vi "PI_Line_Scan_Prepare.vi"(0 "Pixel":u16=100, 3 "Line Length":dbl=20.0 min=0.1 max=200.0 format="%1.1f um", 5 "Wave Cycles":u16, 7 "Axis":enum32{"x-Axis", "y-Axis", "z-Axis"}(ring), 9 "Scanner Divider":i32) -> (14 "Commandset out":string[](array[string]), 16 "Measurement time / [s]":dbl)   [LabVIEW 2011]
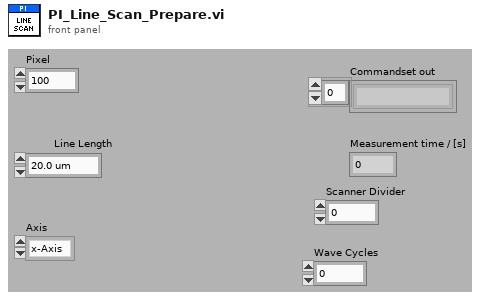
[diagram p1: front panel]
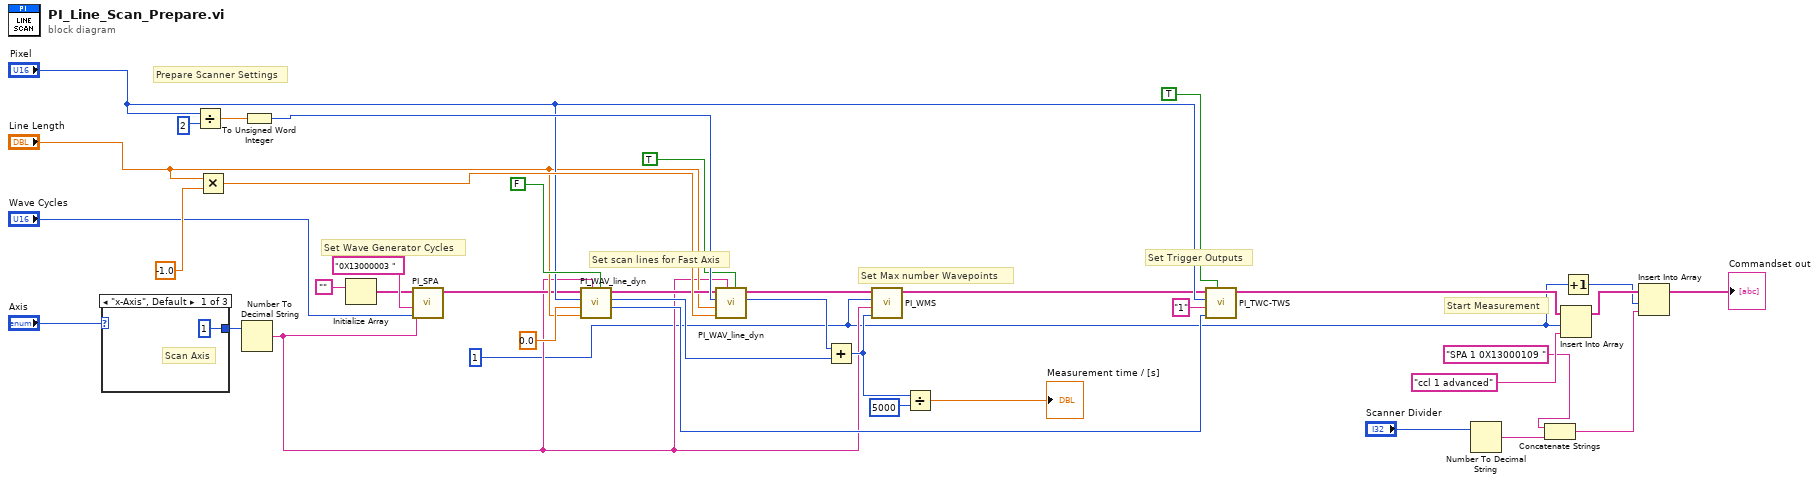
[diagram p0: block diagram]
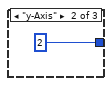
[diagram p2: hidden frame]
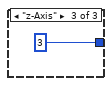
[diagram p3: hidden frame]
diagram:
  w7 = 1 ("Position / Commandset")
  # "Set Wave Generator Cycles"
  # "Start Measurement"
  # "Set Trigger Outputs"
  # "Set Max number Wavepoints"
  # "Set scan lines for Fast Axis"
  # "Prepare Scanner Settings"
  n1 = case shown="\"x-Axis\", Default" "Axis" {
    tunnel: [1 2 3] -> w27
    frame "x-Axis", Default {
      # "Scan Axis"
    }
    frame "y-Axis" {
    }
    frame "z-Axis" {
    }
  }
  n2 = Divide(x="Pixel", y=u16 2) -> (x/y=w32:dbl)
  n3 = Multiply(x="Line Length", y=-1.0) -> (x*y=w34:dbl)
  n4 = Number To Decimal String(number=w27) -> (decimal integer string=w11:string)  [unwired: 1 out]
  n5 = To Unsigned Word Integer(number=w32) -> (unsigned 16bit integer=w33:u16)
  n6 = Initialize Array("") -> (w3:string[])  [unwired: 1 out]
  n7 = call "PI_SPA.vi"("Value"="Wave Cycles", "Register"="0X13000003 " ("string"), "Axis"=w11, "Commandset in"=w3) -> ("Commandset out"=w14:string[])  [unwired: 7 out]
  n8 = call "PI_WAV_line_dyn.vi"("Attach to wav"=FALSE, "Axis Identifier"=w11, "Amplitude / [mu]"="Line Length", "Startpos / [mu]"=0.0, "Pixel per scan"="Pixel", "Commandset in"=w14) -> ("Curve-Start-Pixel"=w26:u16, "Num_Pix"=w24:u16, "Commandset out"=w29:string[])  [unwired: 3 out]
  n9 = call "PI_WAV_line_dyn.vi"("Attach to wav"=TRUE, "Axis Identifier"=w11, "Amplitude / [mu]"=w34, "Startpos / [mu]"="Line Length", "Pixel per scan"=w33, "Commandset in"=w29) -> ("Num_Pix"=w36:u16, "Commandset out"=w37:string[])  [unwired: 4 out]
  n10 = Add(x=w36, y=w24) -> (x+y=w12:u16)
  n11 = call "PI_WMS.vi"("Pixels to reserve"=w12, "Axis"=w11, "Position / Commandset"=w7, "Commandset in"=w37) -> ("Commandset out"=w13:string[])  [unwired: 7 out]
  n12 = Divide(x=w12, y=5000) -> (x/y=→"Measurement time / [s]":dbl)
  n13 = call "PI_TWC-TWS.vi"("TWC?"=TRUE, "Curve_Start_Pixel"=w26, "Axis Identifier"="1", "Pixel per scan"="Pixel", "Commandset in"=w13) -> ("Commandset out"=w10:string[])  [unwired: 6 out]
  n14 = Number To Decimal String(number="Scanner Divider") -> (decimal integer string=w16:string)  [unwired: 1 in]
  n15 = Concatenate Strings("SPA 1 0X13000109 " ("Neues Element/Teil-Array"), w16) -> (w17:string)
  n16 = Insert Into Array(array=w10, index=w7, new element="ccl 1 advanced" ("Neues Element/Teil-Array")) -> (w20:string[])
  n17 = Increment(x=w7) -> (x+1=w6:i32)
  n18 = Insert Into Array(array=w20, index=w6, new element=w17) -> (→"Commandset out":string[])
